vi "Read Buffer Data from Server.vi"(8 "error in (no error)":errorcluster, 9 "timeout ms (25000)":i32=25000, 11 "server ID in":refnum<k5>) -> (0 "error out":errorcluster, 1 "metrics":T1, 2 "buffer data":string, 3 "server ID out":refnum<k5>, 4 "timed out?":bool)   [LabVIEW 2021, in "DSF Core.lvlib"]
uses:
  DSF Core.lvlib
  Metrics.ctl
  Data Server Thread.lvclass
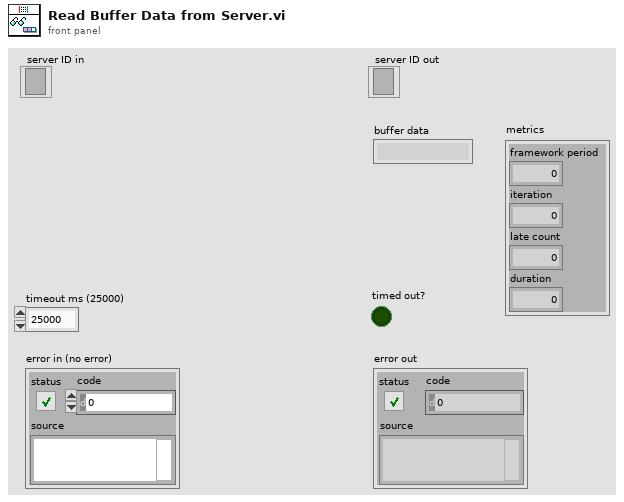
[diagram p1: front panel]
types:
  T1 = typedef "DSF Core.lvlib/Data Server Thread.lvclass/Metrics.ctl" = cluster{"framework period":u32, "iteration":u64, "late count":u64, "duration":u64}
  T2 = enum16{"big-endian, network order", "native, host order", "little-endian"}
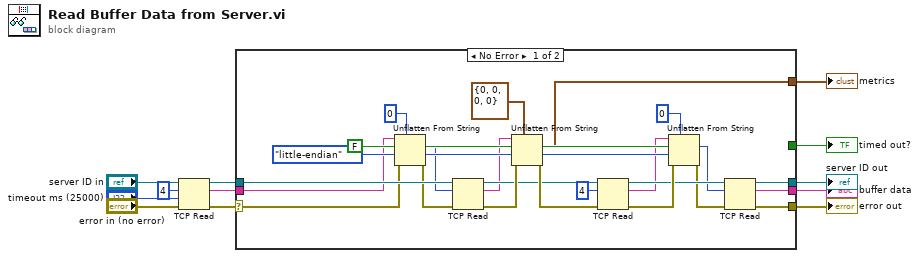
[diagram p0: block diagram]
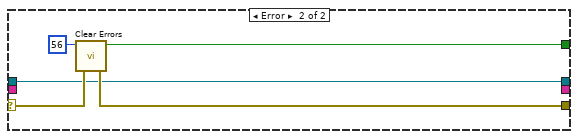
[diagram p2: hidden frame]
diagram:
  n1 = TCP Read(connection ID="server ID in", bytes to read=4, error in (no error)="error in (no error)", 9:"timeout ms (25000)") -> (connection ID out=w8:refnum<k5>, data out=w6:string, error out=w2:errorcluster)  [unwired: 1 in]
  n2 = case shown="No Error" w2 {
    selector: w2 -> [w20 w40]
    tunnel: w8 -> [w36 w38]
    tunnel: [w14 _] -> w7
    tunnel: w6 -> [w13 _]
    tunnel: [w23 _] -> w5
    tunnel: [w22 w38] -> w4
    tunnel: [w21 w39] -> w3
    tunnel: [_ w37] -> w1
    frame No Error {
      w19 = T2."little-endian" ("byte order (0:big-endian, network order)")
      w18 = FALSE ("data includes array or string size? (T)")
      n3 = Unflatten From String(type=0, binary string=w13, data includes array or string size? (T)=w18, byte order (0:big-endian, network order)=w19, error in (no error)=w20) -> (value=w17:i32, error out=w34:errorcluster)  [unwired: 1 out]
      n4 = TCP Read(connection ID=w36, bytes to read=w17, error in (no error)=w34) -> (connection ID out=w25:refnum<k5>, data out=w16:string, error out=w32:errorcluster)  [unwired: 2 in]
      n5 = Unflatten From String(type=T1 {"framework period"=0, "iteration"=0, "late count"=0, "duration"=0} ("metrics"), binary string=w16, data includes array or string size? (T)=w18, byte order (0:big-endian, network order)=w19, error in (no error)=w32) -> (value=w14:T1, error out=w26:errorcluster)  [unwired: 1 out]
      n6 = TCP Read(connection ID=w25, bytes to read=4, error in (no error)=w26) -> (connection ID out=w29:refnum<k5>, data out=w15:string, error out=w31:errorcluster)  [unwired: 2 in]
      n7 = Unflatten From String(type=0, binary string=w15, data includes array or string size? (T)=w18, byte order (0:big-endian, network order)=w19, error in (no error)=w31) -> (value=w24:i32, error out=w27:errorcluster)  [unwired: 1 out]
      n8 = TCP Read(connection ID=w29, bytes to read=w24, error in (no error)=w27) -> (connection ID out=w22:refnum<k5>, data out=w23:string, error out=w21:errorcluster)  [unwired: 2 in]
    }
    frame Error {
      n9 = call <vilib>:"Clear Errors.vi"("error in (no error)"=w40, "specific error code to clear (0: all)"=56) -> ("error out"=w39:errorcluster, "specific error cleared?"=w37:bool)  [unwired: 4 in]
    }
  }
  "error out" <- w3
  "server ID out" <- w4
  "timed out?" <- w1
  "buffer data" <- w5
  "metrics" <- w7
